vi "Convert to Rectangle.vi"(8 "Bottom":i16, 9 "Right":i16, 10 "Top":i16, 11 "Left":i16) -> (3 "Rectangle":T1)   [LabVIEW 2020, in "MacroAssert.lvlib"]
uses:
  MacroAssert.lvlib
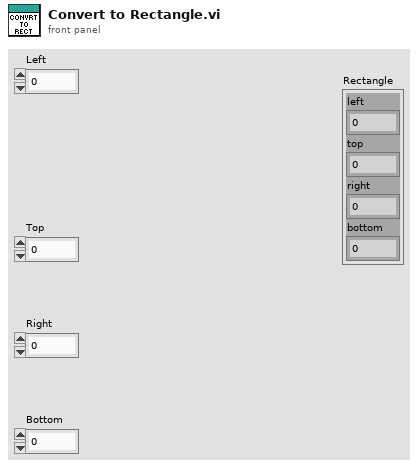
[diagram p1: front panel]
types:
  T1 = cluster{"left":i16, "top":i16, "right":i16, "bottom":i16}
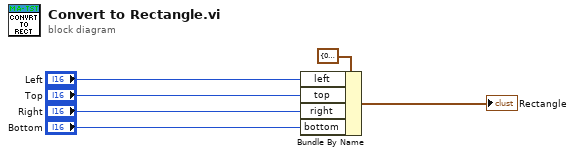
[diagram p0: block diagram]
diagram:
  n1 = Bundle By Name(cluster=T1 {"left"=0, "top"=0, "right"=0, "bottom"=0} ("subset rect"), "left"="Left", "top"="Top", "right"="Right", "bottom"="Bottom") -> (→"Rectangle":T1)
